vi "DeleteOneRecordFrom2DListCtrl.vi"(10 "record index":u16, 11 "ArrayRef in":refnum<vi>) -> (3 "ArrayRef out":refnum<vi>)   [LabVIEW 2018, in "Library-Ctrl.lvlib"]
uses:
  Library-Ctrl.lvlib
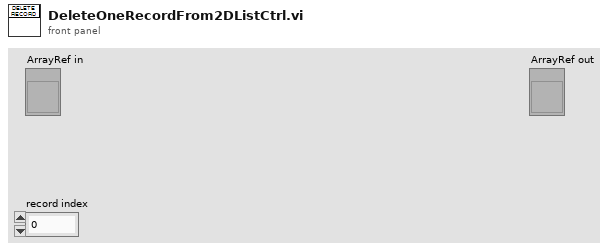
[diagram p1: front panel]
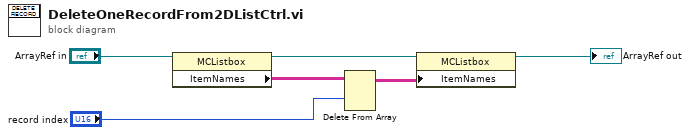
[diagram p0: block diagram]
diagram:
  n1 = property class="MCListbox"(reference="ArrayRef in") -> (reference out=w3:refnum<vi>, "ItemNames"=w5:string[][])  [unwired: 1 in, 1 out]
  n2 = Delete From Array(array=w5, index (row)="record index") -> (array with subset deleted=w2:string[][])  [unwired: 2 in, 1 out]
  n3 = property class="MCListbox"(reference=w3, "ItemNames"=w2) -> (reference out=→"ArrayRef out":refnum<vi>)  [unwired: 1 in, 1 out]
